vi "Advance past comma.vi"(7 "JSON":string, 9 "Offset":i32, 11 "State in":T1=enum."Leading Whitespace") -> (1 "Offset past match":i32, 3 "State":T1=enum."Value end")   [LabVIEW 2013, in "JSONtext.lvlib"]
uses:
  JSONtext.lvlib
  Parsing State.ctl
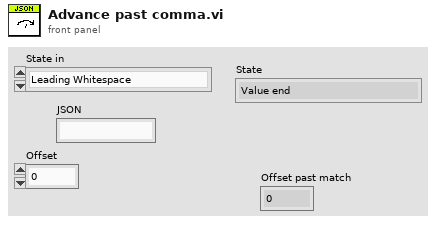
[diagram p1: front panel]
types:
  T1 = typedef "JSONtext.lvlib/Parsing State.ctl" = enum16{"Parser Error", "Object", "Array", "String", "Number/Other", "Leading Whitespace", "Object end", "Array end", "Value end"}
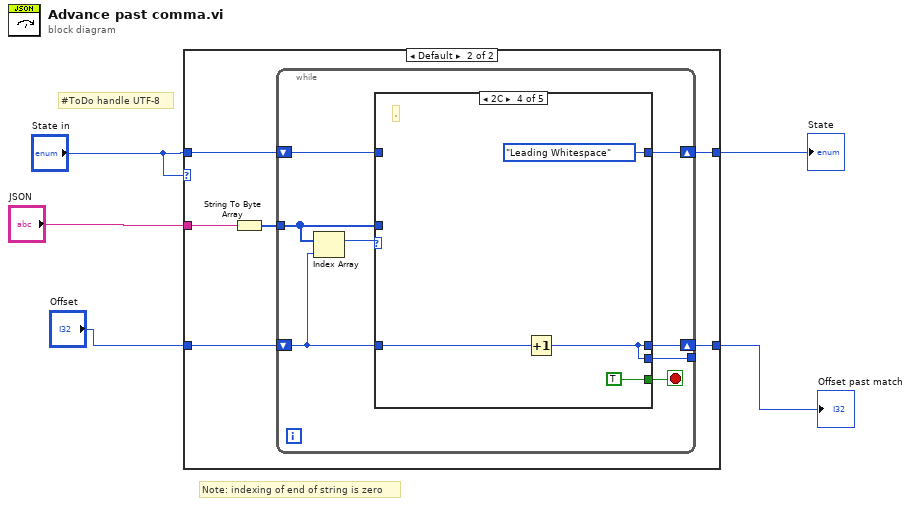
[diagram p0: block diagram]
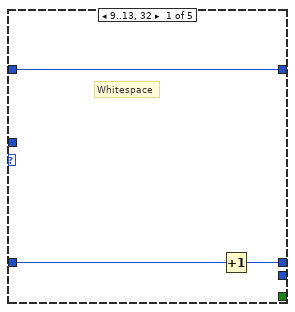
[diagram p3: hidden frame]
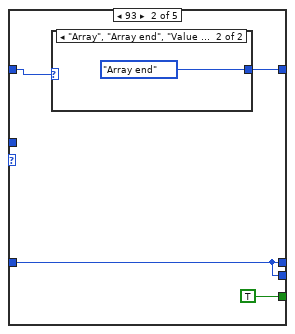
[diagram p4: hidden frame]
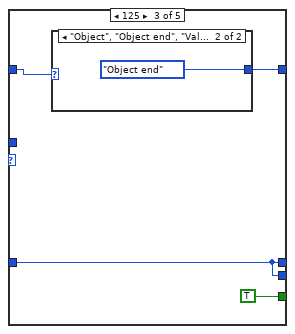
[diagram p6: hidden frame]
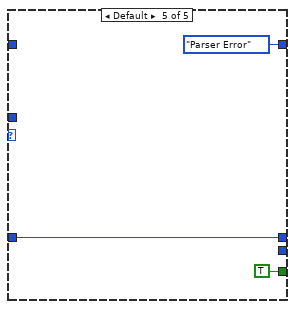
[diagram p8: hidden frame]
diagram:
  # "Note: indexing of end of string is zero"
  # "#ToDo handle UTF-8"
  n1 = case shown="Default" "State in" {
    tunnel: [w7 w13] -> w5
    tunnel: [w6 w12] -> w4
    tunnel: "State in" -> [w7 w11]
    tunnel: "Offset" -> [w6 w8]
    tunnel: "JSON" -> [_ w9]
    frame "Parser Error" {
    }
    frame Default {
      n2 = String To Byte Array(string=w9) -> (unsigned byte array=w10:u8[])
      n3 = while {
        tunnel: w10 -> [w20]
        shift-right: [w15] -> w12
        shift-left: w8 -> [w16]
        shift-right: [w18] -> w13
        shift-left: w11 -> [w19]
        tunnel: [w14] -> _
        stop <- w17 stop-if-true
        n4 = Index Array(array=w20, index=w16) -> (element=w21:u8)
        n5 = case shown="2C" w21 {
          tunnel: w20 -> [_ _ _ _ _]
          tunnel: w19 -> [w24 w25 w30 _ _]
          tunnel: [w24 w28 w33 Parsing_State."Leading Whitespace" Parsing_State."Parser Error"] -> w18
          tunnel: [_ TRUE TRUE TRUE TRUE] -> w17
          tunnel: w16 -> [w23 w26 w31 w37 w41]
          tunnel: [w22 w26 w31 w35 w41] -> w15
          tunnel: [_ w26 w31 w35 _] -> w14
          frame 9..13, 32 {
            # "Whitespace"
            n6 = Increment(x=w23) -> (x+1=w22:i32)
          }
          frame 93 {
            n7 = case shown="\"Array\", \"Array end\", \"Value end\"" w25 {
              tunnel: [_ Parsing_State."Array end"] -> w28
              frame Default {
              }
              frame "Array", "Array end", "Value end" {
              }
            }
          }
          frame 125 {
            n8 = case shown="\"Object\", \"Object end\", \"Value end\"" w30 {
              tunnel: [_ Parsing_State."Object end"] -> w33
              frame Default {
              }
              frame "Object", "Object end", "Value end" {
              }
            }
          }
          frame 44 {
            # ","
            n9 = Increment(x=w37) -> (x+1=w35:i32)
          }
          frame Default {
          }
        }
      }
    }
  }
  "State" <- w5
  "Offset past match" <- w4
